vi "Show Pane Settings UI.vi"(8 "Error In":errorcluster, 10 "Pane":refnum<class "Pane.lvclass">, 11 "Pane Settings UI in":refnum<class "Pane Settings UI.lvclass">) -> (0 "Error Out":errorcluster, 3 "Pane Settings UI out":refnum<class "Pane Settings UI.lvclass">)   [LabVIEW 2015, in "Pane Settings UI.lvlib" / "Pane Settings UI.lvclass"]
uses:
  Pane Settings UI.lvclass
  Classes/Pane/Pane.lvclass
  <vilib>/ActorFramework/Actor/Actor.lvclass/Actor.ctl
  <vilib>/ActorFramework/Message Enqueuer/Message Enqueuer.lvclass/Message Enqueuer.ctl
  Pane Settings UI.lvclass/Pane Settings UI.ctl
  <vilib>/ActorFramework/Message Enqueuer/Init from Existing Queue.vi
  <vilib>/ActorFramework/Message Enqueuer/Message Enqueuer.lvclass
  <vilib>/MGI/Panel Manager/Panel Actor/Panel Actor Messages/Show Panel Msg/Show Panel Msg.lvclass
  <vilib>/ActorFramework/Actor/Actor.lvclass
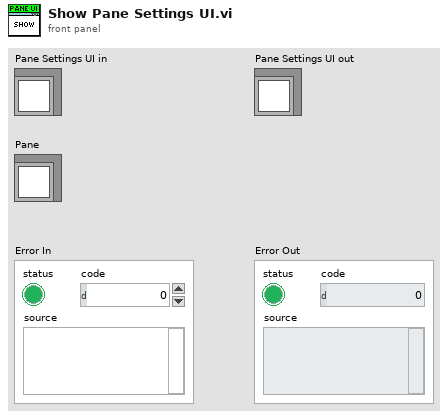
[diagram p1: front panel]
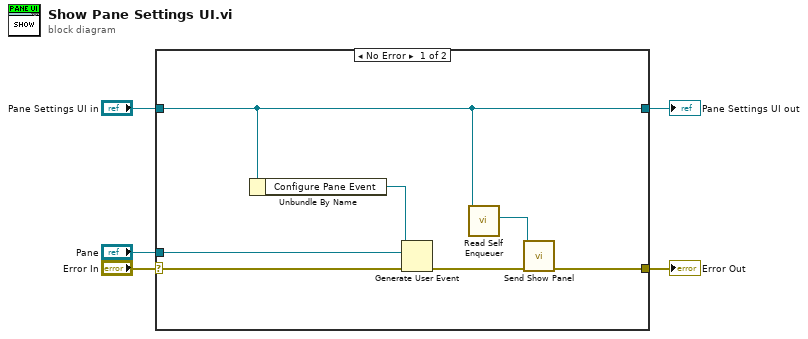
[diagram p0: block diagram]
diagram:
  n1 = case shown="No Error" "Error In" {
    selector: "Error In" -> [w8 w14]
    tunnel: [w6 w14] -> w2
    tunnel: [w7 w13] -> w4
    tunnel: "Pane Settings UI in" -> [w7 w13]
    tunnel: "Pane" -> [w9 _]
    frame No Error {
      n2 = Unbundle By Name(w7) -> ("Configure Pane Event"=w12:refnum<user-event>)
      n3 = Generate User Event(user event=w12, event data cluster=w9, error in=w8) -> (error out=w11:errorcluster)  [unwired: 1 in, 1 out]
      n4 = call <vilib>:"Read Self Enqueuer.vi"("Actor"=w7) -> ("Self Enqueuer"=w10:refnum<class "Message Enqueuer.lvclass">)  [unwired: 10 in]
      n5 = call <vilib>:"Send Show Panel.vi"("Error In"=w11, "Message Enqueuer in"=w10) -> ("Error Out"=w6:errorcluster)  [unwired: 8 in, 1 out]
    }
    frame Error {
    }
  }
  "Pane Settings UI out" <- w4
  "Error Out" <- w2
